vi "MPM_Set_Logging_Paremeter_for_STS.vi"(0 ".NET Reference in":refnum<k24>, 1 "startwave":dbl, 2 "stopwave":dbl, 3 "wavestep":dbl, 4 "speed":dbl, 5 "error in (no error)":errorcluster, 6 "acctualstep":dbl, 7 "mode":i32(ring) items=["ManualRangeConstant", "ManualRangeSweep", "AutoRangeConstant", "AutoRangeSweep", "Freerun"]) -> (14 "Reference out":refnum<k24>, 19 "error out":errorcluster)   [LabVIEW 2017]
doc: "Sweep parameter setting"
uses:
  D:/test/PDLSTS/LV_PDL LvVer17.0/LV_PDL_x64/DLL/InstrumentDLL.dll
  DLL/InstrumentDLL.dll
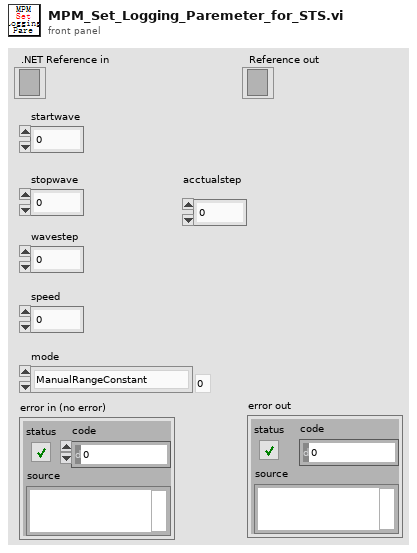
[diagram p1: front panel]
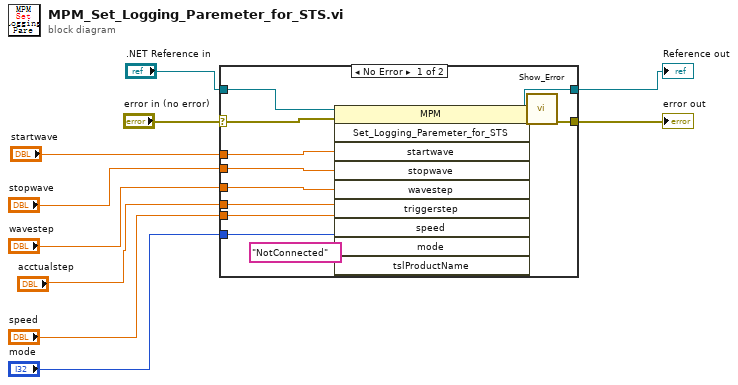
[diagram p0: block diagram]
diagram:
  n1 = case shown="No Error" "error in (no error)" {
    selector: "error in (no error)" -> [w21 w24]
    tunnel: ".NET Reference in" -> [w23 w25]
    tunnel: [w22 w25] -> w9
    tunnel: [w20 w24] -> w7
    tunnel: "startwave" -> [w17 _]
    tunnel: "stopwave" -> [w16 _]
    tunnel: "wavestep" -> [w15 _]
    tunnel: "speed" -> [w12 _]
    tunnel: "mode" -> [w13 _]
    tunnel: "acctualstep" -> [w11 _]
    frame No Error {
      n2 = invoke class="MPM" method="Set_Logging_Paremeter_for_STS"(reference=w23, error in=w21, "startwave"=w17, "stopwave"=w16, "wavestep"=w15, "triggerstep"=w11, "speed"=w12, "mode"=w13, "tslProductName"="NotConnected") -> (reference out=w22:refnum<k24>, error out=w19:errorcluster, "Set_Logging_Paremeter_for_STS"=w18:i32)  [unwired: 1 in, 7 out]
      n3 = call "Show_Error.vi"("error in (no error)"=w19, "Error"=w18) -> ("error out"=w20:errorcluster)  [unwired: 9 in]
    }
    frame Error {
    }
  }
  "Reference out" <- w9
  "error out" <- w7
